vi "get_Photoelectron_scaling.vi"(8 "error in (no error)":errorcluster, 11 "Hamamatsu_C9100-13 in":refnum<class "Hamamatsu_C9100-13.lvclass">) -> (0 "error out":errorcluster, 2 "Photoelectron Scaling":dbl=5.8, 3 "Hamamatsu_C9100-13 out":refnum<class "Hamamatsu_C9100-13.lvclass">)   [LabVIEW 2013]
uses:
  Hamamatsu_C9100-13.lvclass
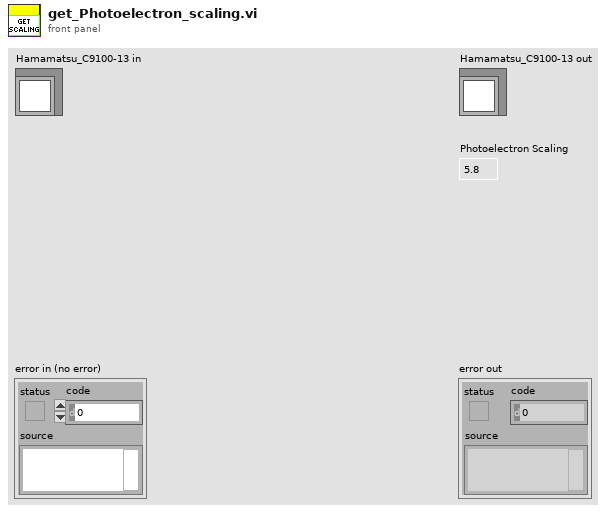
[diagram p1: front panel]
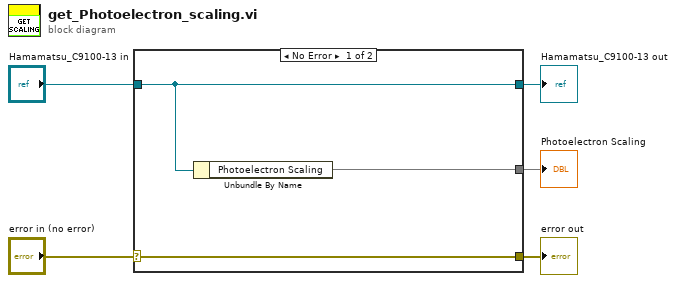
[diagram p0: block diagram]
diagram:
  n1 = case shown="No Error" "error in (no error)" {
    selector: "error in (no error)" -> [w8 w9]
    tunnel: [w8 w9] -> w4
    tunnel: [w7 w10] -> w2
    tunnel: "Hamamatsu_C9100-13 in" -> [w7 w10]
    tunnel: [w6 _] -> w1
    frame No Error {
      n2 = Unbundle By Name(w7) -> ("Photoelectron Scaling"=w6)
    }
    frame Error {
    }
  }
  "error out" <- w4
  "Hamamatsu_C9100-13 out" <- w2
  "Photoelectron Scaling" <- w1
